vi "PanelSetting.vi"() -> ()   [LabVIEW 2014]
uses:
  <vilib>/userdefined/High Color/IMAQdx.ctl
panel:
  in  "UpCamTool":refnum<vi>
  in  "CalibBoard_Project_Path":path
  in  "Session In":T1
  in  "UpScale":dbl
  out "Current Position":refnum<vi>
  in  "Btn_Exist":refnum<vi>
  in  "InsertPanel?":bool
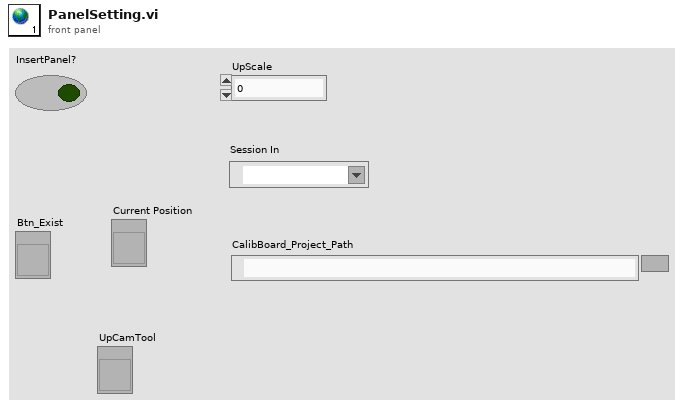
[diagram p1: front panel]
types:
  T1 = typedef "IMAQdx.ctl" = refnum<k21>
diagram:
